vi "Initialize Keithley DMM.vi"(8 "error in (no error)":errorcluster, 11 "DMM":refnum<visa-resource-name>="DMM") -> (0 "error out":errorcluster, 3 "DMM out":refnum<visa-resource-name>)   [LabVIEW 2015]
uses:
  <instrlib>/Keithley 27XX/Keithley 27XX.lvlib
panel:
  in  "Serial Configuration":T1={"Baud Rate (19200)"=19200, "Flow Control (1: XON/XOFF)"=1, "Termination Char (0:CR)"=0} {"Termination Char (0:CR)" items=["CR", "LF"]; "Flow Control (1: XON/XOFF)" items=["None", "XON/XOFF", "RTS/CTS (2701 Only)", "XON/XOFF & RTS/CTS (2701 Only)"]; "Baud Rate (19200)" items=["300"=300, "600"=600, "1200"=1200, "2400"=2400, "4800"=4800, "9600"=9600, "19.2k"=19200, "38.4k (2701 Only)"=38400, "57.6k (2701 Only)"=57600, "115.2k (2701 Only)"=115200]}
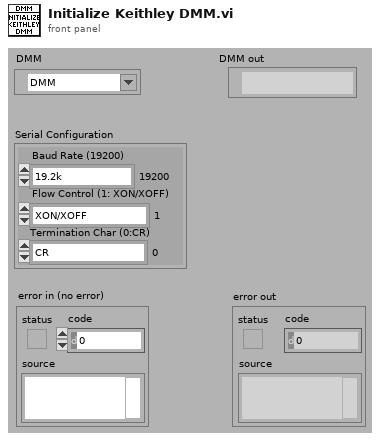
[diagram p1: front panel]
types:
  T1 = cluster{"Baud Rate (19200)":u32, "Flow Control (1: XON/XOFF)":u16, "Termination Char (0:CR)":u16}
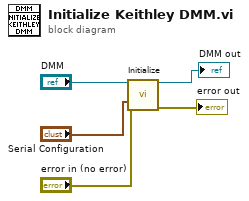
[diagram p0: block diagram]
diagram:
  n1 = call <instrlib>:"Initialize.vi"("VISA resource name"="DMM", "Serial Configuration"="Serial Configuration", "error in (no error)"="error in (no error)") -> ("VISA resource name out"=→"DMM out":refnum<visa-resource-name>, "error out"=→"error out":errorcluster)  [unwired: 11 in]
